vi "SelectProductModel.vi"(8 "error in (no error)":errorcluster, 11 "TestBench in":refnum<class "TestBench.lvclass">) -> (0 "error out":errorcluster, 3 "TestBench out":refnum<class "TestBench.lvclass">)   [LabVIEW 2019, in "TestBench.lvlib" / "TestBench.lvclass"]
uses:
  TestBench.lvclass
  TestBench.lvclass/TestBench.ctl
  TestSetup/TestSetup Messages/Write TestLimitPath Msg/Write TestLimitPath Msg.lvclass/Write TestLimitPath Msg.ctl
  <vilib>/ActorFramework/Message Enqueuer/Message Enqueuer.lvclass/Message Enqueuer.ctl
  <vilib>/ActorFramework/Message Enqueuer/Enqueue.vi
  TestSetup/TestSetup Messages/Write TestLimitPath Msg/Write TestLimitPath Msg.lvclass
  C:/Program Files (x86)/National Instruments/LabVIEW 2019/vi.lib/ActorFramework/Message/Message.lvclass
  <vilib>/ActorFramework/Message Priority Queue/Priority Enqueue.vi
panel:
  in  "OK":bool
  in  "Cancel":bool
  in  "ProductModel":string(combo)
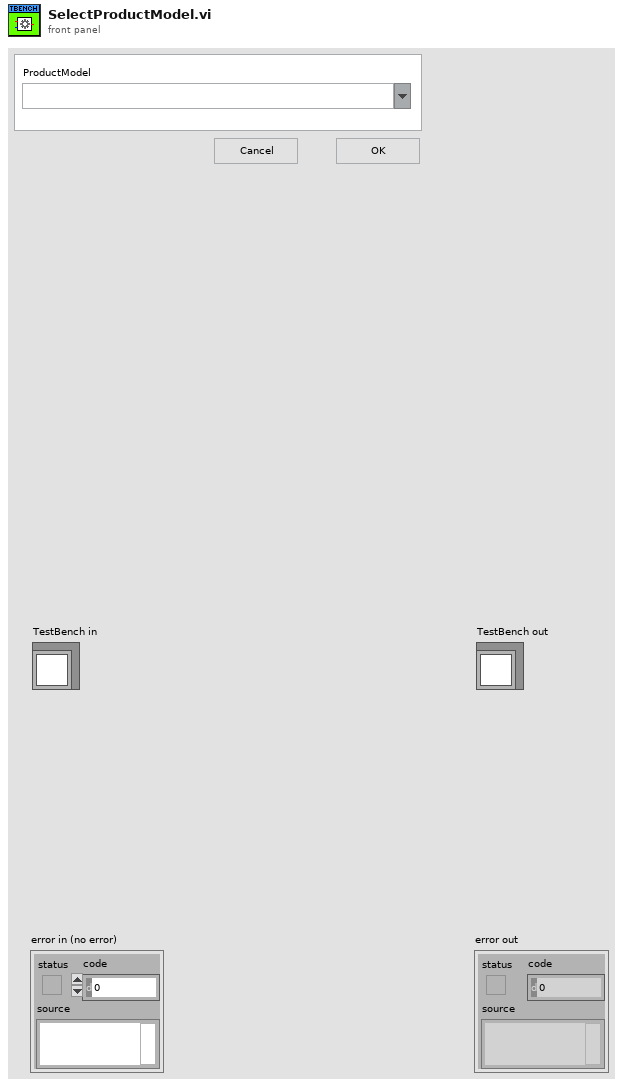
[diagram p1: front panel]
types:
  T1 = enum32{"Invalid", "Standard", "Closed", "Hidden", "Minimized", "Maximized"}
  T2 = enum32{"invalid app kind", "Development System", "Run Time System", "Student Edition", "Embedded LabVIEW", "Evaluation", "Custom"}
  T3 = cluster{"Core":cluster{"Current VI Reference":refnum<vi>, "Close Panel on Exit?":bool}, "ProductModel":refnum<vi>}
  T4 = cluster{"Current VI Reference":refnum<vi>, "Close Panel on Exit?":bool}
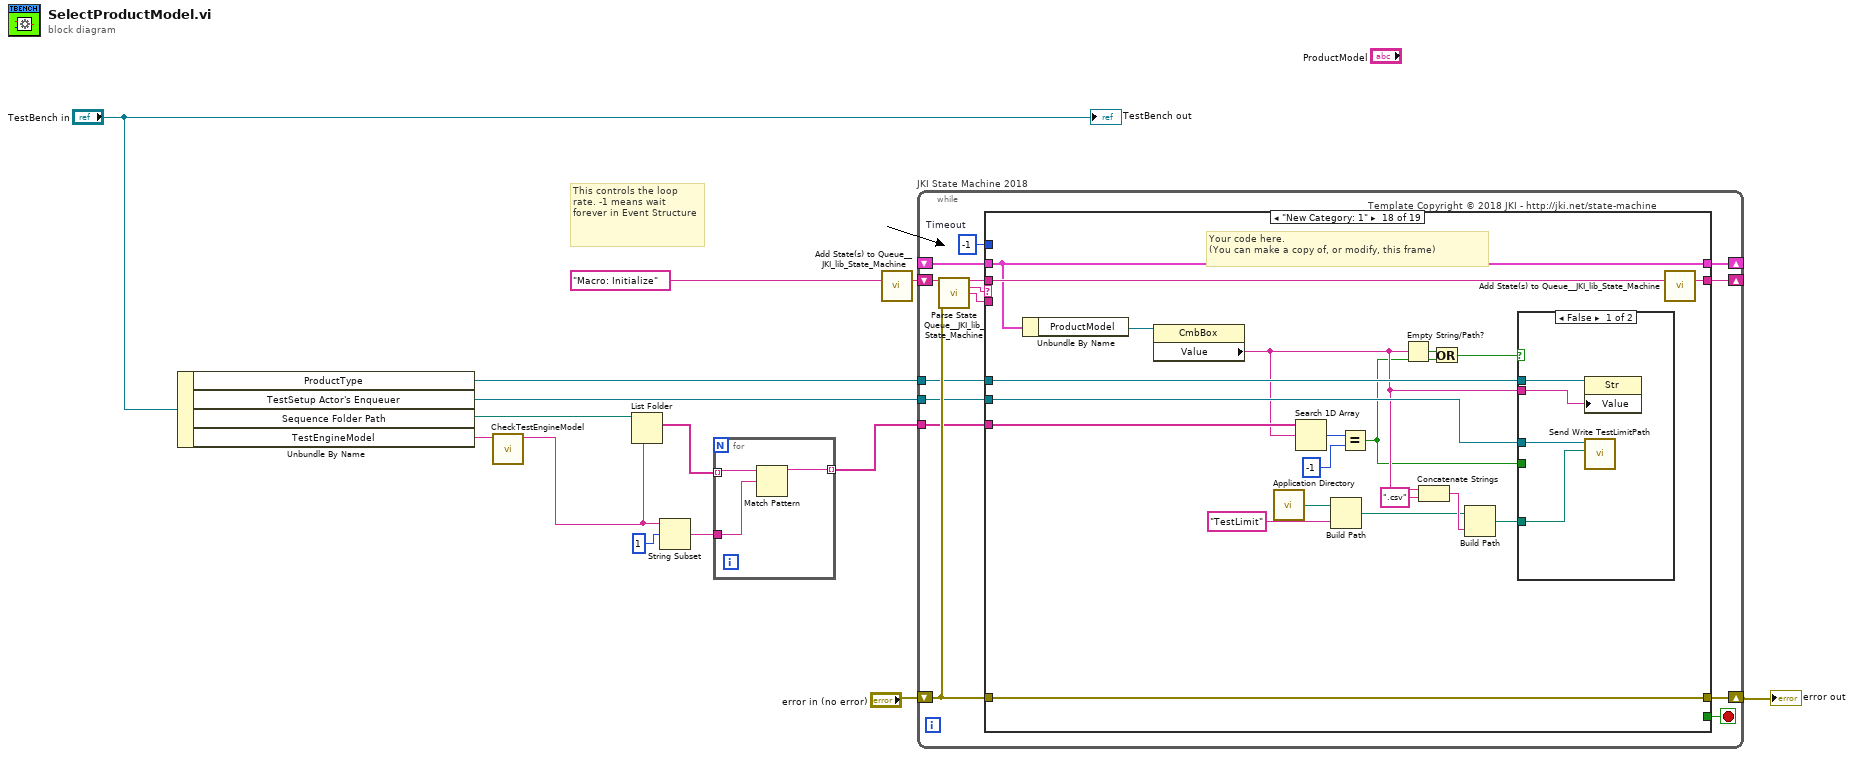
[diagram p0: block diagram]
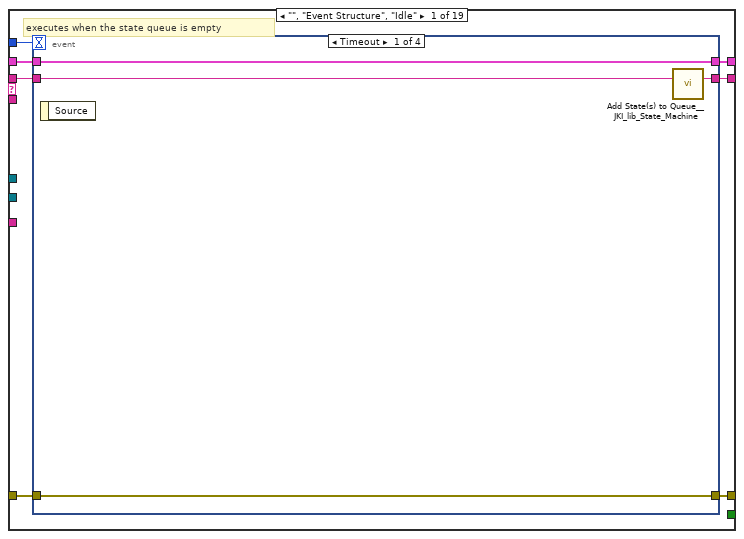
[diagram p2: hidden frame]
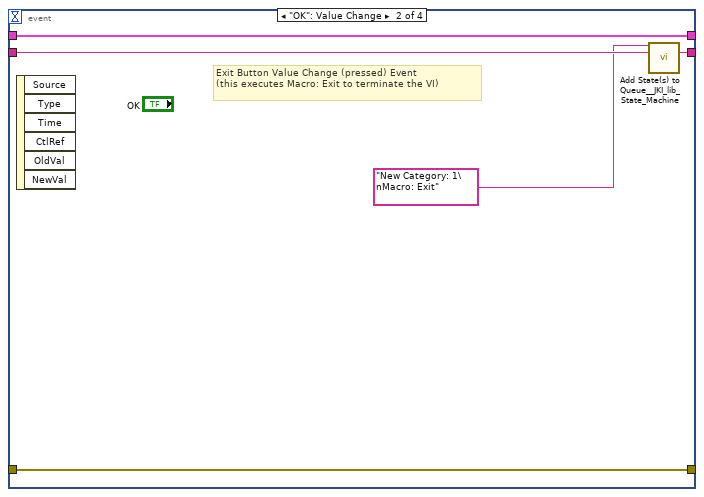
[diagram p3: hidden frame]
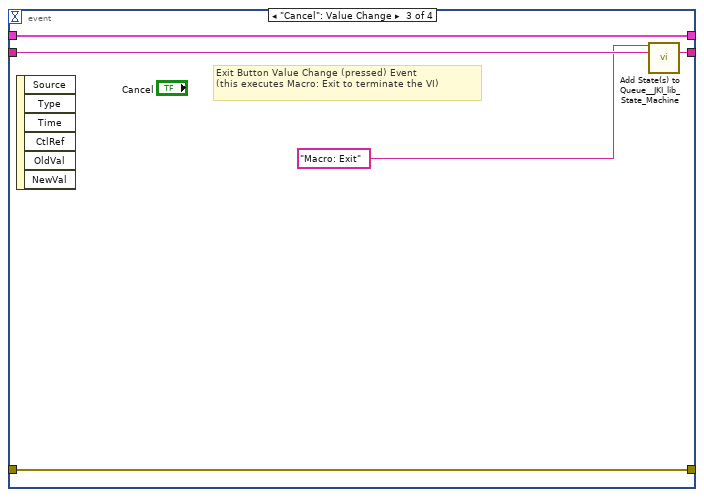
[diagram p4: hidden frame]
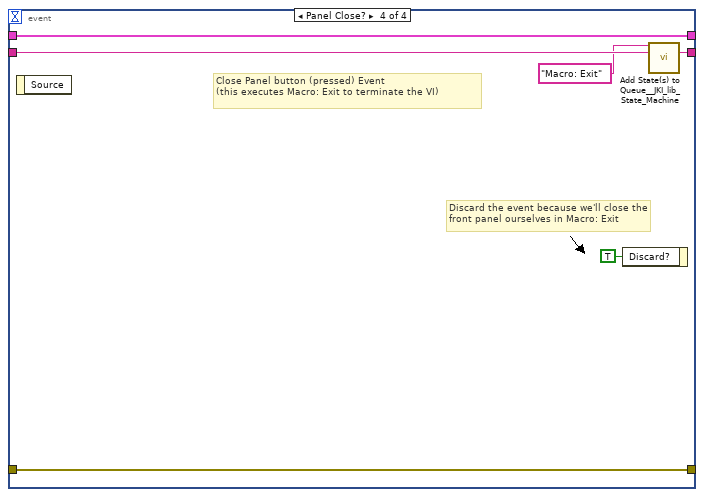
[diagram p5: hidden frame]
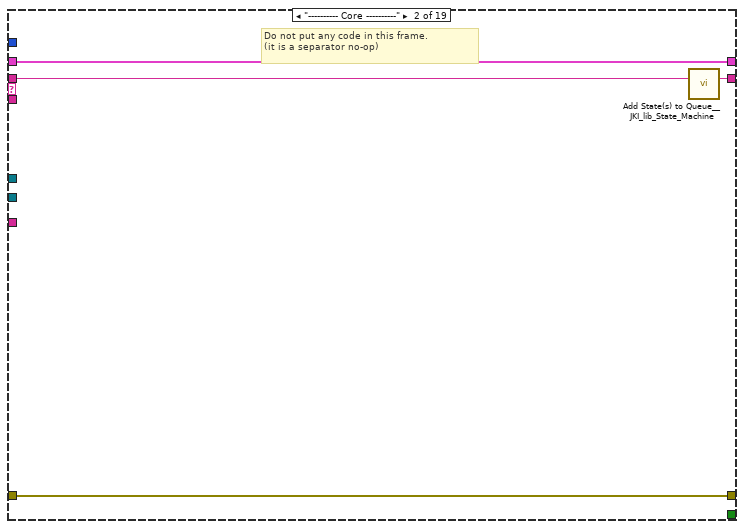
[diagram p6: hidden frame]
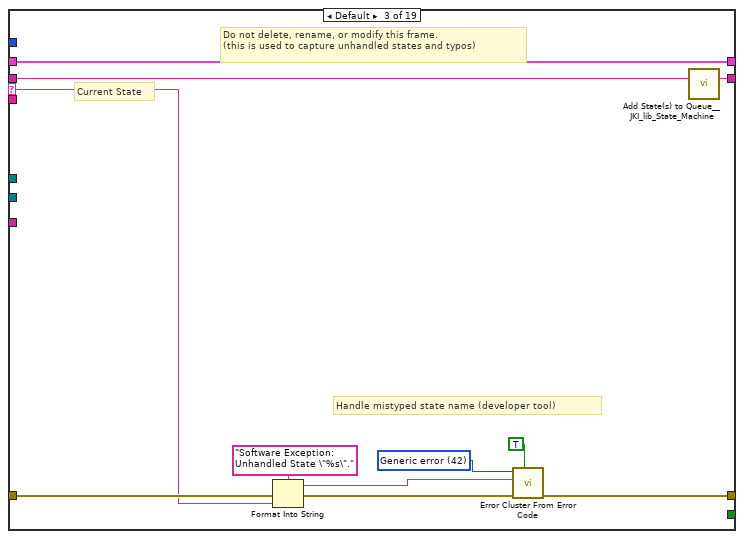
[diagram p7: hidden frame]
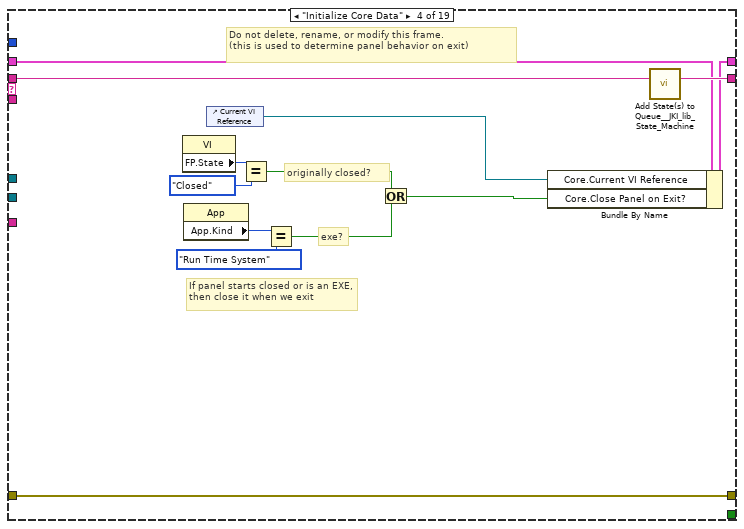
[diagram p8: hidden frame]
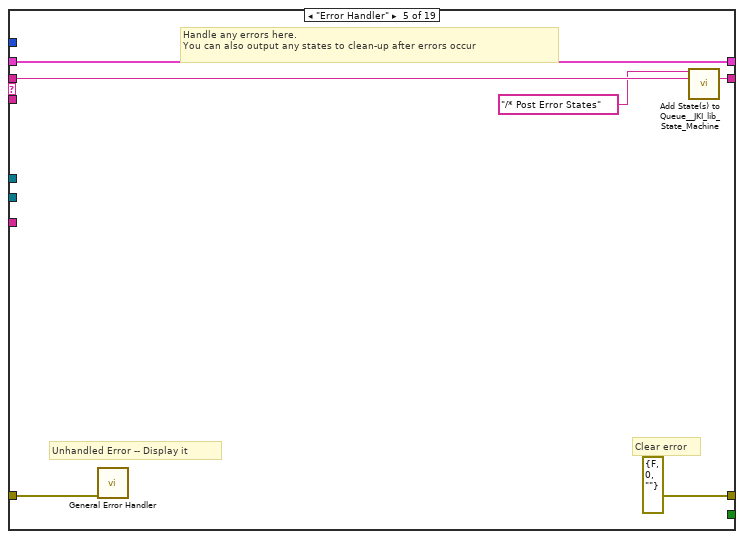
[diagram p9: hidden frame]
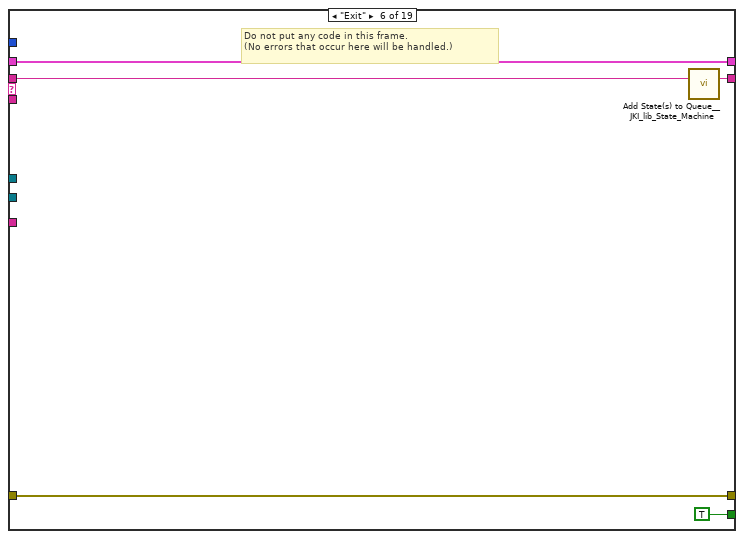
[diagram p10: hidden frame]
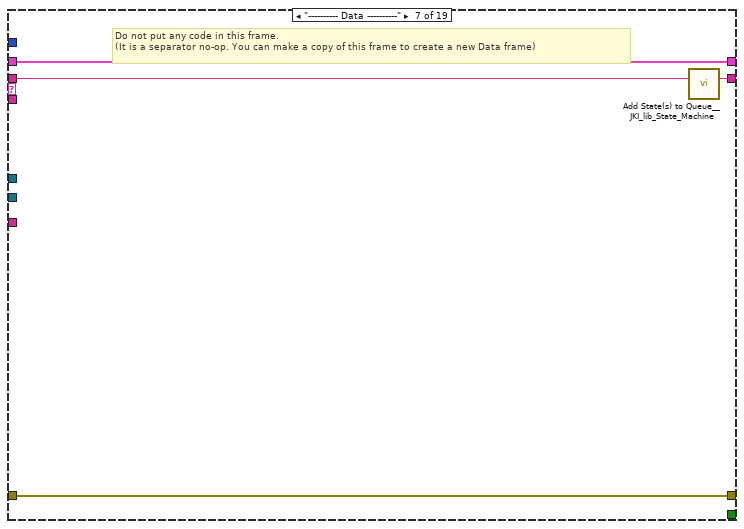
[diagram p11: hidden frame]
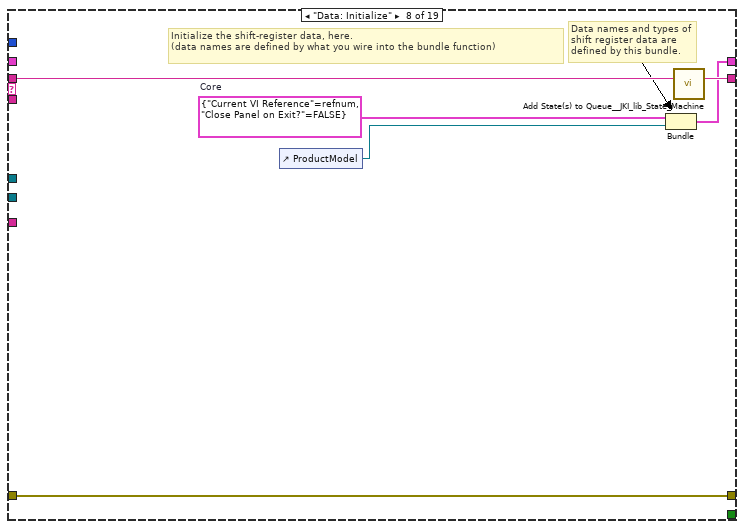
[diagram p12: hidden frame]
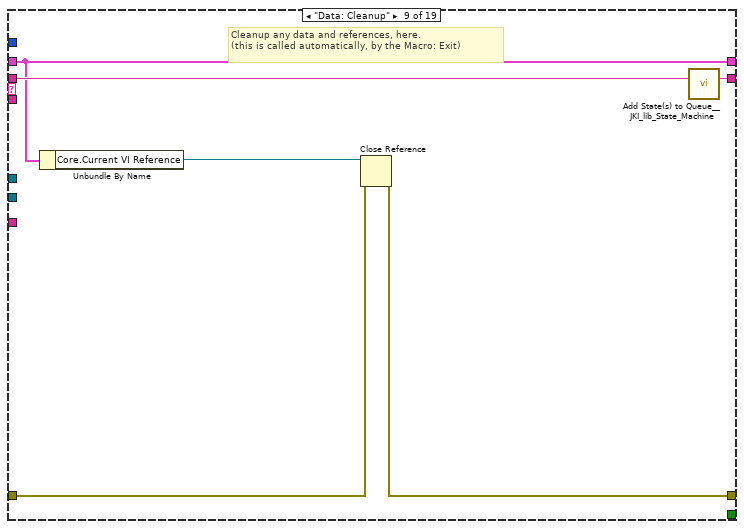
[diagram p13: hidden frame]
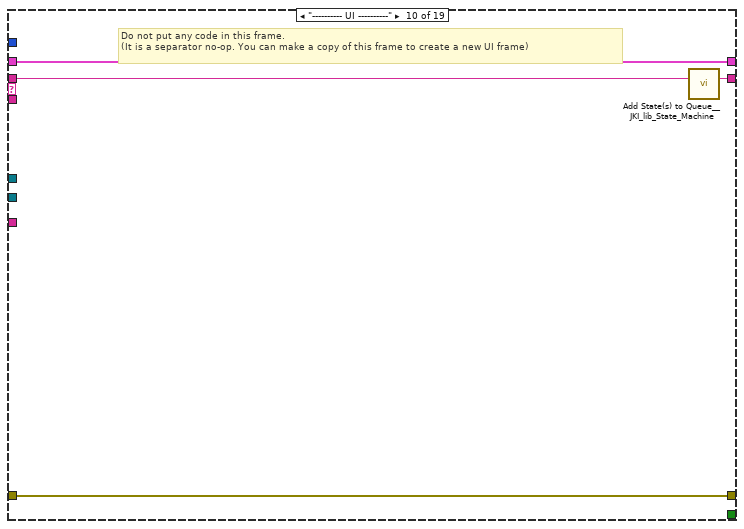
[diagram p14: hidden frame]
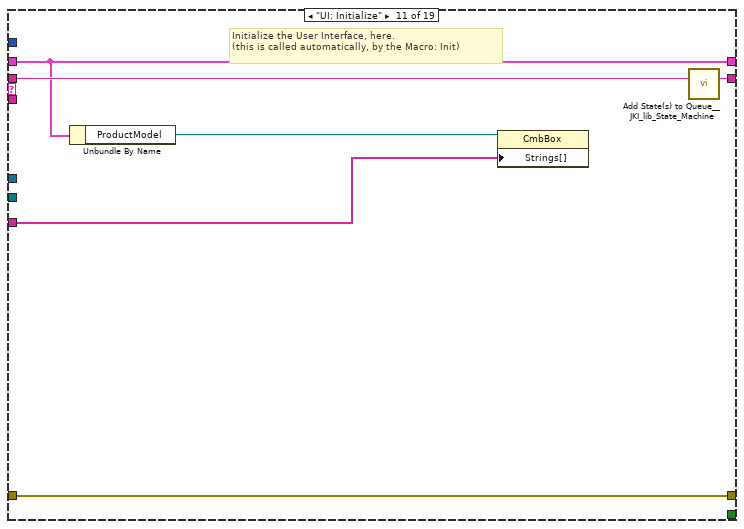
[diagram p15: hidden frame]
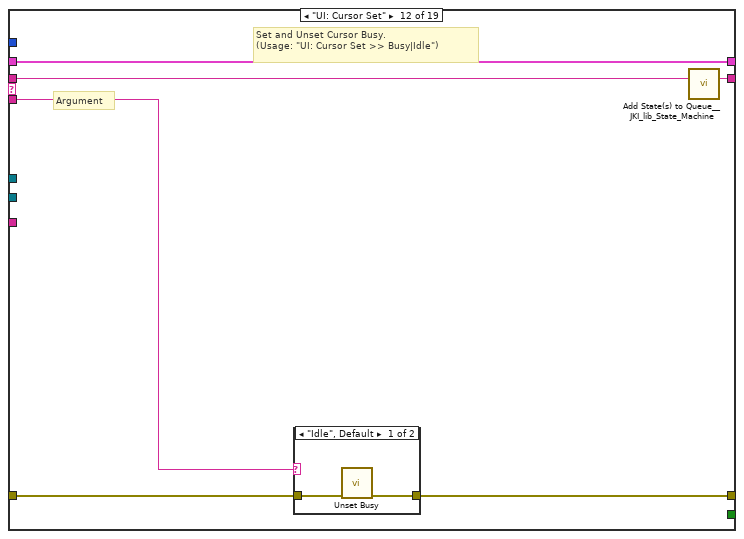
[diagram p16: hidden frame]
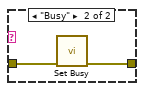
[diagram p17: hidden frame]
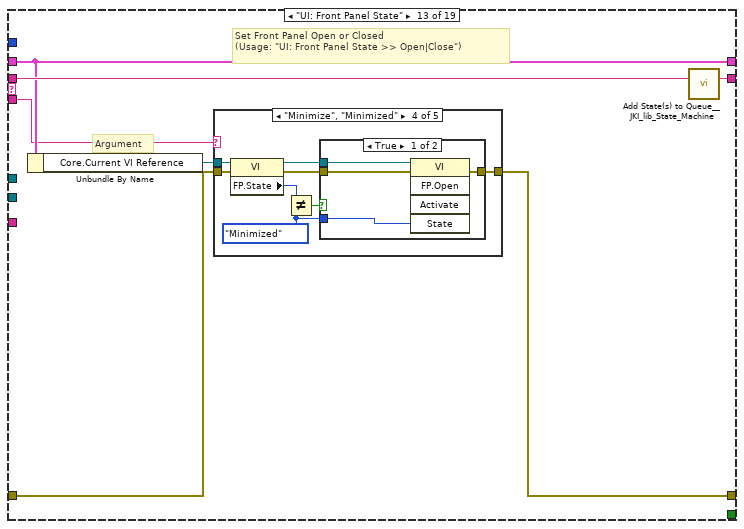
[diagram p18: hidden frame]
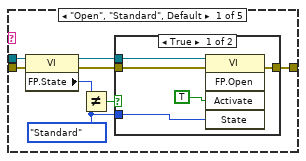
[diagram p19: hidden frame]
diagram:
  # "This controls the loop rate. -1 means wait forever in Event Structure"
  n1 = Unbundle By Name("TestBench in") -> ("ProductType"=w8:refnum<vi>, "TestSetup Actor's Enqueuer"=w9:refnum<class "Message Enqueuer.lvclass">, "Sequence Folder Path"=w7:path, "TestEngineModel"=w2:string)
  n2 = call "CheckTestEngineModel.vi"("Modle"=w2) -> ("Pattern"=w1:string)  [unwired: 10 in]
  n3 = List Folder(path=w7, pattern=w1) -> (filenames=w6:string[])  [unwired: 2 in, 3 out]
  n4 = String Subset(string=w1, offset (0)=1) -> (substring=w3:string)  [unwired: 1 in]
  n5 = for {
    tunnel: w6 -> [w17] mode=indexing
    tunnel: [w16] -> w5 mode=indexing
    tunnel: w3 -> [w15]
    n6 = Match Pattern(string=w17, regular expression=w15) -> (before substring=w16:string)  [unwired: 1 in, 3 out]
  }
  n7 = call <vilib>:"Add State(s) to Queue__JKI_lib_State_Machine.vi"("State(s) in (\"\")"="Macro: Initialize") -> ("States Out"=w14:string)  [unwired: 14 in]
  n8 = while "JKI State Machine 2018" {
    shift-right: [w24] -> _
    shift-left: _ -> [w23]
    shift-right: [w27] -> w11
    shift-left: "error in (no error)" -> [w21]
    shift-right: [w26] -> _
    shift-left: w14 -> [w28]
    tunnel: w9 -> [w20]
    tunnel: w8 -> [w19]
    tunnel: w5 -> [w18]
    stop <- w25 stop-if-true
    w22 = -1  # Timeout
    # "Template Copyright © 2018 JKI - http://jki.net/state-machine"
    n9 = call <vilib>:"Parse State Queue__JKI_lib_State_Machine.vi"("State Queue"=w28, "Error In (no error)"=w21) -> ("Remaining States"=w30:string, "Current State"=w31:string, "Arguments"=w29:string)  [unwired: 11 in]
    n10 = case shown="\"New Category: 1\"" w31 {
      selector: w31 -> [_ _ w63 _ _ _ _ _ _ _ _ _ _ _ _ _ _ _ _]
      tunnel: w30 -> [w38 w62 w67 w86 w92 w97 w101 w107 w113 w117 w123 w129 w140 w209 w214 w224 w228 w248 w258]
      tunnel: w29 -> [_ _ _ _ _ _ _ _ _ _ _ w124 w134 _ _ _ _ _ _]
      tunnel: w23 -> [w36 w59 w65 w79 w89 w95 w98 _ w108 w114 w120 w127 w136 w206 w211 w221 w225 w245 w255]
      tunnel: [w35 w60 w69 w83 errorcluster {"status"=FALSE, "code"=0, "source"=""} ("error out") w94 w99 w104 w109 w115 w121 w125 w137 w207 w212 w222 w226 w246 w256] -> w27
      tunnel: w21 -> [w34 w60 w68 w83 w88 w94 w99 w104 w110 w115 w121 w126 w138 w207 w212 w222 w226 w246 w256]
      tunnel: [w37 w61 w66 w85 w91 w96 w100 w106 w112 w116 w122 w128 w139 w208 w213 w223 w227 w247 w257] -> w26
      tunnel: [_ _ _ _ _ TRUE _ _ _ _ _ _ _ _ _ _ _ _ _] -> w25
      tunnel: [w33 w59 w65 w84 w89 w95 w98 w105 w108 w114 w120 w127 w136 w206 w211 w221 w225 w245 w255] -> w24
      tunnel: w22 -> [w32 _ _ _ _ _ _ _ _ _ _ _ _ _ _ _ _ _ _]
      tunnel: w20 -> [_ _ _ _ _ _ _ _ _ _ _ _ _ _ _ _ _ w235 _]
      tunnel: w19 -> [_ _ _ _ _ _ _ _ _ _ _ _ _ _ _ _ _ w243 _]
      tunnel: w18 -> [_ _ _ _ _ _ _ _ _ _ w118 _ _ _ _ _ _ w234 _]
      frame "", "Event Structure", "Idle" {
        # "executes when the state queue is empty"
        n11 = event shown="[0] Timeout" {
          selector: _ -> [_ _ _ _]
          dyn-events: _ -> [_ _ _ _]
          timeout: w32 -> [_ _ _ _]
          tunnel: w38 -> [w42 w47 w52 w58]
          tunnel: [w41 w46 w51 w57] -> w37
          tunnel: w36 -> [w39 w44 w49 w55]
          tunnel: [w40 w45 w50 w56] -> w35
          tunnel: w34 -> [w40 w45 w50 w56]
          tunnel: [w39 w44 w49 w55] -> w33
          event Timeout {
            n12 = event-data() -> ()  [unwired: 1 in, 1 out]
            n13 = call <vilib>:"Add State(s) to Queue__JKI_lib_State_Machine.vi"("State(s) in (\"\")"=w42) -> ("States Out"=w41:string)  [unwired: 14 in]
          }
          event "OK": Value Change {
            # "Exit Button Value Change (pressed) Event\n(this executes Macro: Exit to terminate the VI)"
            n14 = event-data() -> ()  [unwired: 1 in, 6 out]
            n15 = call <vilib>:"Add State(s) to Queue__JKI_lib_State_Machine.vi"("State(s) in Front (\"\")"="New Category: 1\nMacro: Exit", "State(s) in (\"\")"=w47) -> ("States Out"=w46:string)  [unwired: 13 in]
          }
          event "Cancel": Value Change {
            # "Exit Button Value Change (pressed) Event\n(this executes Macro: Exit to terminate the VI)"
            n16 = event-data() -> ()  [unwired: 1 in, 6 out]
            n17 = call <vilib>:"Add State(s) to Queue__JKI_lib_State_Machine.vi"("State(s) in Front (\"\")"="Macro: Exit", "State(s) in (\"\")"=w52) -> ("States Out"=w51:string)  [unwired: 13 in]
          }
          event Panel Close? {
            # "Discard the event because we'll close the front panel ourselves in Macro: Exit"
            # "Close Panel button (pressed) Event\n(this executes Macro: Exit to terminate the VI)"
            n18 = event-data() -> ()  [unwired: 1 in, 1 out]
            n19 = event-data("Discard?"=TRUE) -> ()  [unwired: 1 in, 1 out]
            n20 = call <vilib>:"Add State(s) to Queue__JKI_lib_State_Machine.vi"("State(s) in Front (\"\")"="Macro: Exit", "State(s) in (\"\")"=w58) -> ("States Out"=w57:string)  [unwired: 13 in]
          }
        }
      }
      frame "---------- Core ----------" {
        # "Do not put any code in this frame.\n(it is a separator no-op)"
        n21 = call <vilib>:"Add State(s) to Queue__JKI_lib_State_Machine.vi"("State(s) in (\"\")"=w62) -> ("States Out"=w61:string)  [unwired: 14 in]
      }
      frame Default {
        w72 = 42 items=["No error", "Argument error", "Memory is full", "Out of zone", "End of file", "File already open", "Generic file I/O error", "File not found", "File permission error", "Disk is full", "Duplicate path", "Too many files open", "System feature not enabled", "Resource file not found", "Cannot add resource", "Resource not found", "Image not found", "Image memory error", "Pen does not exist", "Config type invalid", "Config token not found", "Config parse error", "Config memory error", "Bad external code format", "Bad external code offset", "External code not present", "Null window", "Destroy window error", "Null menu", "Print aborted", "Bad print record", "Print driver error", "Windows error during printing", "Memory error during printing", "Print dialog error", "Generic print error", "Invalid device refnum", "Device not found", "Device parameter error", "Device unit error", "Cannot open device", "Device call aborted", "Generic error", "Cancelled by user", "Object ID too low", "Object ID too high", "Object not in heap", "Unknown heap", "Unknown object (invalid DefProc)", "Unknown object (DefProc not in table)", "Message out of range", "Invalid (null) method", "Unknown message", "Manager call not supported", "Bad address", "Network operation in progress", "Network operation timed out", "Connection is busy", "Network attribute not supported", "Network error", "Address in use", "System out of memory", "Connection aborted", "Connection refused", "Not connected", "Already connected", "Connection closed", "Initialization error (interapplication manager)", "Bad occurrence", "Wait on unbound occurrence handler", "Occurrence queue overflow", "Datalog type conflict", "Unused", "Unrecognized type (interapplication manager)", "Memory corrupt", "Failed to make temporary DLL", "Old CIN version", "Drag socket not found", "Failed to load drop-object", "Failed to register OLE object", "Failed to release OLE object", "Format specifier type mismatch", "Unknown format specifier", "Too few format specifiers", "Too many format specifiers", "Scan failed", "Newer CIN version", "Error converting to variant", "Runtime menu error", "Password tampered", "Variant attribute not found", "Incompatible variant data type", "Event data is not available", "Event Store is not present", "Occurrence is not found", "Event Queue is not created", "Event info is not available", "Refnum passed is NULL", "Error retrieving Class GUID", "Error retrieving CoClass GUID", "Error retrieving TypeLib GUID.", "Bad built application magic bytes.", "Specific driver is different from the specific driver associated with the Logical Name.", "There is no session opened to the class driver.", "Max Error", "MAX - Error with config objects", "MAX - Error loading configuration", "MAX - Group not supported"]
        # "Current State"
        # "Do not delete, rename, or modify this frame.\n(this is used to capture unhandled states and typos)"
        # "Handle mistyped state name (developer tool)"
        n22 = Format Into String(format string="Software Exception: Unhandled State \"%s\"." ("message"), error in=w68, w63) -> (resulting string=w71:string, error out=w70:errorcluster)  [unwired: 1 in]
        n23 = call <vilib>:"Error Cluster From Error Code.vi"("show call chain? (False)"=TRUE, "error in (no error)"=w70, "error message (\"\")"=w71, "error code (0)"=w72) -> ("error out"=w69:errorcluster)  [unwired: 5 in]
        n24 = call <vilib>:"Add State(s) to Queue__JKI_lib_State_Machine.vi"("State(s) in (\"\")"=w67) -> ("States Out"=w66:string)  [unwired: 14 in]
      }
      frame "Initialize Core Data" {
        # "Do not delete, rename, or modify this frame.\n(this is used to determine panel behavior on exit)"
        # "originally closed?"
        # "exe?"
        # "If panel starts closed or is an EXE, then close it when we exit"
        n25 = property class="VI"() -> ("FP.State"=w76:T1)  [unwired: 2 in, 2 out]
        n26 = property class="App"() -> ("App.Kind"=w82:T2)  [unwired: 2 in, 2 out]
        n27 = control-ref of="Current VI Reference"() -> (w77:refnum<vi>)
        n28 = Equal?(x=w76, y=T1."Closed" ("Front Panel Window:State")) -> (x = y?=w74:bool)
        n29 = Equal?(x=w82, y=T2."Run Time System" ("Application:Kind")) -> (x = y?=w80:bool)
        n30 = Or(x=w74, y=w80) -> (x .or. y?=w78:bool)
        n31 = Bundle By Name(cluster=w79, "Core.Current VI Reference"=w77, "Core.Close Panel on Exit?"=w78) -> (w84:T3)
        n32 = call <vilib>:"Add State(s) to Queue__JKI_lib_State_Machine.vi"("State(s) in (\"\")"=w86) -> ("States Out"=w85:string)  [unwired: 14 in]
      }
      frame "Error Handler" {
        # "Unhandled Error -- Display it"
        # "Handle any errors here.\nYou can also output any states to clean-up after errors occur"
        # "Clear error"
        n33 = call <vilib>:"General Error Handler.vi"("error in (no error)"=w88) -> ()  [unwired: 10 in, 5 out]
        n34 = call <vilib>:"Add State(s) to Queue__JKI_lib_State_Machine.vi"("State(s) in Front (\"\")"="/* Post Error States", "State(s) in (\"\")"=w92) -> ("States Out"=w91:string)  [unwired: 13 in]
      }
      frame "Exit" {
        # "Do not put any code in this frame.\n(No errors that occur here will be handled.)"
        n35 = call <vilib>:"Add State(s) to Queue__JKI_lib_State_Machine.vi"("State(s) in (\"\")"=w97) -> ("States Out"=w96:string)  [unwired: 14 in]
      }
      frame "---------- Data ----------" {
        # "Do not put any code in this frame.\n(It is a separator no-op. You can make a copy of this frame to create a new Data frame)"
        n36 = call <vilib>:"Add State(s) to Queue__JKI_lib_State_Machine.vi"("State(s) in (\"\")"=w101) -> ("States Out"=w100:string)  [unwired: 14 in]
      }
      frame "Data: Initialize" {
        w103 = T4 {"Current VI Reference"=refnum, "Close Panel on Exit?"=FALSE}  # Core
        # "Data names and types of shift register data are defined by this bundle."
        # "Initialize the shift-register data, here.\n(data names are defined by what you wire into the bundle function)"
        n37 = control-ref of="ProductModel"() -> (w102:refnum<vi>)
        n38 = Bundle("Core"=w103, "ProductModel"=w102) -> (w105:T3)  [unwired: 1 in]
        n39 = call <vilib>:"Add State(s) to Queue__JKI_lib_State_Machine.vi"("State(s) in (\"\")"=w107) -> ("States Out"=w106:string)  [unwired: 14 in]
      }
      frame "Data: Cleanup" {
        # "Cleanup any data and references, here.\n(this is called automatically, by the Macro: Exit)"
        n40 = Unbundle By Name(w108) -> ("Core.Current VI Reference"=w111:refnum<vi>)
        n41 = Close Reference(reference=w111, error in (no error)=w110) -> (error out=w109:errorcluster)
        n42 = call <vilib>:"Add State(s) to Queue__JKI_lib_State_Machine.vi"("State(s) in (\"\")"=w113) -> ("States Out"=w112:string)  [unwired: 14 in]
      }
      frame "---------- UI ----------" {
        # "Do not put any code in this frame.\n(It is a separator no-op. You can make a copy of this frame to create a new UI frame)"
        n43 = call <vilib>:"Add State(s) to Queue__JKI_lib_State_Machine.vi"("State(s) in (\"\")"=w117) -> ("States Out"=w116:string)  [unwired: 14 in]
      }
      frame "UI: Initialize" {
        # "Initialize the User Interface, here.\n(this is called automatically, by the Macro: Init)"
        n44 = Unbundle By Name(w120) -> ("ProductModel"=w119:refnum<vi>)
        n45 = property class="CmbBox"(reference=w119, "Strings[]"=w118) -> ()  [unwired: 1 in, 2 out]
        n46 = call <vilib>:"Add State(s) to Queue__JKI_lib_State_Machine.vi"("State(s) in (\"\")"=w123) -> ("States Out"=w122:string)  [unwired: 14 in]
      }
      frame "UI: Cursor Set" {
        # "Argument"
        # "Set and Unset Cursor Busy.\n(Usage: \"UI: Cursor Set >> Busy|Idle\")"
        n47 = case shown="\"Idle\", Default" w124 {
          tunnel: w126 -> [w131 w133]
          tunnel: [w130 w132] -> w125
          frame "Idle", Default {
            n48 = call <vilib>:"Unset Busy.vi"("error in (no error)"=w131) -> ("error out"=w130:errorcluster)  [unwired: 10 in]
          }
          frame "Busy" {
            n49 = call <vilib>:"Set Busy.vi"("error in (no error)"=w133) -> ("error out"=w132:errorcluster)  [unwired: 9 in, 1 out]
          }
        }
        n50 = call <vilib>:"Add State(s) to Queue__JKI_lib_State_Machine.vi"("State(s) in (\"\")"=w129) -> ("States Out"=w128:string)  [unwired: 14 in]
      }
      frame "UI: Front Panel State" {
        # "Argument"
        # "Set Front Panel Open or Closed\n(Usage: \"UI: Front Panel State >> Open|Close\")"
        n51 = Unbundle By Name(w136) -> ("Core.Current VI Reference"=w135:refnum<vi>)
        n52 = case shown="\"Minimize\", \"Minimized\"" w134 {
          tunnel: w138 -> [w146 w161 w172 w185 w198]
          tunnel: [w148 w162 w174 w187 w200] -> w137
          tunnel: w135 -> [w147 w159 w173 w186 w199]
          frame "Open", "Standard", Default {
            w141 = T1."Standard" ("State")
            n53 = property class="VI"(reference=w147, error in=w146) -> (reference out=w144:refnum<vi>, error out=w145:errorcluster, "FP.State"=w143:T1)
            n54 = Not Equal?(x=w143, y=w141) -> (x != y?=w142:bool)
            n55 = case shown="True" w142 {
              tunnel: [w152 w154] -> w148
              tunnel: w145 -> [w151 w154]
              tunnel: w144 -> [w150 _]
              tunnel: w141 -> [w149 _]
              frame True {
                n56 = invoke class="VI" method="FP.Open"(reference=w150, error in=w151, "Activate"=TRUE, "State"=w149) -> (error out=w152:errorcluster)  [unwired: 1 in, 4 out]
              }
              frame False {
              }
            }
          }
          frame "Close", "Closed" {
            n57 = property class="VI"(reference=w159, error in=w161) -> (reference out=w158:refnum<vi>, error out=w160:errorcluster, "FP.State"=w156:T1)
            n58 = Not Equal?(x=w156, y=T1."Closed" ("Front Panel Window:State")) -> (x != y?=w155:bool)
            n59 = case shown="True" w155 {
              tunnel: [w163 w166] -> w162
              tunnel: w160 -> [w163 w165]
              tunnel: w158 -> [_ w164]
              frame False {
              }
              frame True {
                n60 = invoke class="VI" method="FP.Close"(reference=w164, error in=w165) -> (error out=w166:errorcluster)  [unwired: 1 in, 2 out]
              }
            }
          }
          frame "Hidden", "Hide" {
            w167 = T1."Hidden" ("State")
            n61 = property class="VI"(reference=w173, error in=w172) -> (reference out=w170:refnum<vi>, error out=w171:errorcluster, "FP.State"=w169:T1)
            n62 = Not Equal?(x=w169, y=w167) -> (x != y?=w168:bool)
            n63 = case shown="True" w168 {
              tunnel: [w178 w179] -> w174
              tunnel: w171 -> [w177 w179]
              tunnel: w170 -> [w176 _]
              tunnel: w167 -> [w175 _]
              frame True {
                n64 = invoke class="VI" method="FP.Open"(reference=w176, error in=w177, "State"=w175) -> (error out=w178:errorcluster)  [unwired: 2 in, 4 out]
              }
              frame False {
              }
            }
          }
          frame "Minimize", "Minimized" {
            w180 = T1."Minimized" ("State")
            n65 = property class="VI"(reference=w186, error in=w185) -> (reference out=w183:refnum<vi>, error out=w184:errorcluster, "FP.State"=w182:T1)
            n66 = Not Equal?(x=w182, y=w180) -> (x != y?=w181:bool)
            n67 = case shown="True" w181 {
              tunnel: [w191 w192] -> w187
              tunnel: w184 -> [w190 w192]
              tunnel: w183 -> [w189 _]
              tunnel: w180 -> [w188 _]
              frame True {
                n68 = invoke class="VI" method="FP.Open"(reference=w189, error in=w190, "State"=w188) -> (error out=w191:errorcluster)  [unwired: 2 in, 4 out]
              }
              frame False {
              }
            }
          }
          frame "Maximize", "Maximized" {
            w193 = T1."Maximized" ("State")
            n69 = property class="VI"(reference=w199, error in=w198) -> (reference out=w196:refnum<vi>, error out=w197:errorcluster, "FP.State"=w195:T1)
            n70 = Not Equal?(x=w195, y=w193) -> (x != y?=w194:bool)
            n71 = case shown="True" w194 {
              tunnel: [w204 w205] -> w200
              tunnel: w197 -> [w203 w205]
              tunnel: w196 -> [w202 _]
              tunnel: w193 -> [w201 _]
              frame True {
                n72 = invoke class="VI" method="FP.Open"(reference=w202, error in=w203, "State"=w201) -> (error out=w204:errorcluster)  [unwired: 2 in, 4 out]
              }
              frame False {
              }
            }
          }
        }
        n73 = call <vilib>:"Add State(s) to Queue__JKI_lib_State_Machine.vi"("State(s) in (\"\")"=w140) -> ("States Out"=w139:string)  [unwired: 14 in]
      }
      frame "---------- Macro ----------" {
        # "Do not put any code in this frame.\n(It is a separator no-op. You can make a copy of this frame to create a new Macro frame)"
        n74 = call <vilib>:"Add State(s) to Queue__JKI_lib_State_Machine.vi"("State(s) in (\"\")"=w209) -> ("States Out"=w208:string)  [unwired: 14 in]
      }
      frame "Macro: Initialize" {
        w210 = "Data: Initialize\nInitialize Core Data\nUI: Initialize\nUI: Front Panel State >> Open"  # Data: Initialize Initialize Core Data UI: Initialize UI: Front Panel State >> Open
        # "Initialization Macro\n(This is called once, when the VI starts)"
        n75 = call <vilib>:"Add State(s) to Queue__JKI_lib_State_Machine.vi"("State(s) in Front (\"\")"=w210, "State(s) in (\"\")"=w214) -> ("States Out"=w213:string)  [unwired: 13 in]
      }
      frame "Macro: Exit" {
        # "Exit Macro\n(This is called once, when the VI exits)"
        n76 = Unbundle By Name(w221) -> ("Core.Close Panel on Exit?"=w220:bool)
        n77 = Select(t="UI: Front Panel State >> Close", s=w220, f="") -> (s? t:f=w217:string)
        n78 = call <vilib>:"Add State(s) to Queue__JKI_lib_State_Machine.vi"("State(s) in (\"\")"=w217, "State(s) at Back (\"\")"="Data: Cleanup\nExit") -> ("States Out"=w215:string)  [unwired: 13 in]
        n79 = call <vilib>:"Add State(s) to Queue__JKI_lib_State_Machine.vi"("State(s) in Front (\"\")"=w215, "State(s) in (\"\")"=w224) -> ("States Out"=w223:string)  [unwired: 13 in]
      }
      frame "---------- New Category ----------" {
        # "Template Separator\n(You can make a copy of, or modify, this frame)"
        n80 = call <vilib>:"Add State(s) to Queue__JKI_lib_State_Machine.vi"("State(s) in (\"\")"=w228) -> ("States Out"=w227:string)  [unwired: 14 in]
      }
      frame "New Category: 1" {
        # "Your code here.\n(You can make a copy of, or modify, this frame)"
        n81 = Unbundle By Name(w245) -> ("ProductModel"=w244:refnum<vi>)
        n82 = property class="CmbBox"(reference=w244) -> ("Value"=w233:string)  [unwired: 1 in, 2 out]
        n83 = call <vilib>:"Application Directory.vi"() -> ("Application Directory"=w240:path)
        n84 = Search 1D Array(1D array=w234, element=w233) -> (index of element=w232:i32)  [unwired: 1 in]
        n85 = Build Path(base path=w240, name or relative path="TestLimit") -> (appended path=w237:path)
        n86 = Equal?(x=w232, y=-1) -> (x = y?=w229:bool)
        n87 = Empty String/Path?(string/path=w233) -> (empty?=w242:bool)
        n88 = Concatenate Strings(w233, ".csv" ("string")) -> (w238:string)
        n89 = Or(x=w242, y=w229) -> (x .or. y?=w230:bool)
        n90 = Build Path(base path=w237, name or relative path=w238) -> (appended path=w236:path)
        n91 = case shown="False" w230 {
          tunnel: w243 -> [w252 _]
          tunnel: w233 -> [w251 _]
          tunnel: w236 -> [w249 _]
          tunnel: w235 -> [w250 _]
          tunnel: w229 -> [_ w253]
          frame False {
            n92 = property class="Str"(reference=w252, "Value"=w251) -> ()  [unwired: 1 in, 2 out]
            n93 = call "Send Write TestLimitPath.vi"("TestLimitPath"=w249, "Message Enqueuer"=w250) -> ()  [unwired: 8 in, 2 out]
          }
          frame True {
            n94 = case shown="False" w253 {
              frame False {
              }
              frame True {
                n95 = One Button Dialog(message="Sequence file does not exist , Please confirm again ") -> ()  [unwired: 1 in, 1 out]
              }
            }
          }
        }
        n96 = call <vilib>:"Add State(s) to Queue__JKI_lib_State_Machine.vi"("State(s) in (\"\")"=w248) -> ("States Out"=w247:string)  [unwired: 14 in]
      }
      frame "New Category: 2" {
        # "Your code here.\n(You can make a copy of, or modify, this frame)"
        n97 = call <vilib>:"Add State(s) to Queue__JKI_lib_State_Machine.vi"("State(s) in (\"\")"=w258) -> ("States Out"=w257:string)  [unwired: 14 in]
      }
    }
  }
  "error out" <- w11
  "TestBench out" <- "TestBench in"
